vi "DAC trigger.vi"() -> ()   [LabVIEW 2020]
uses:
  <vilib>/DAQmx/configure/timing.llb/DAQmx Timing (Implicit).vi
  <resource>/objmgr/daqmx.rc
  <vilib>/DAQmx/create/channels.llb/DAQmx Create Channel (AO-Voltage-Basic).vi
  <vilib>/Utility/file.llb/Read Delimited Spreadsheet (DBL).vi
  <vilib>/DAQmx/write.llb/DAQmx Write (Analog 1D DBL 1Chan NSamp).vi
  <vilib>/DAQmx/configure/timing.llb/DAQmx Timing (Sample Clock).vi
  <vilib>/DAQmx/create/channels.llb/DAQmx Create Channel (CO-Pulse Generation-Frequency).vi
panel:
  out "Numeric":i32
  in  "Add flyback to polynomial":dbl[](graph)=array[10000 elements]
  in  "File to read":path=path "C:/Users/Hannah/Downloads/newcalibration_voice coil input_25msflyback.txt"
  out "# Samples written per channel":u32=1000
  out "actual frequency":dbl=1000.0
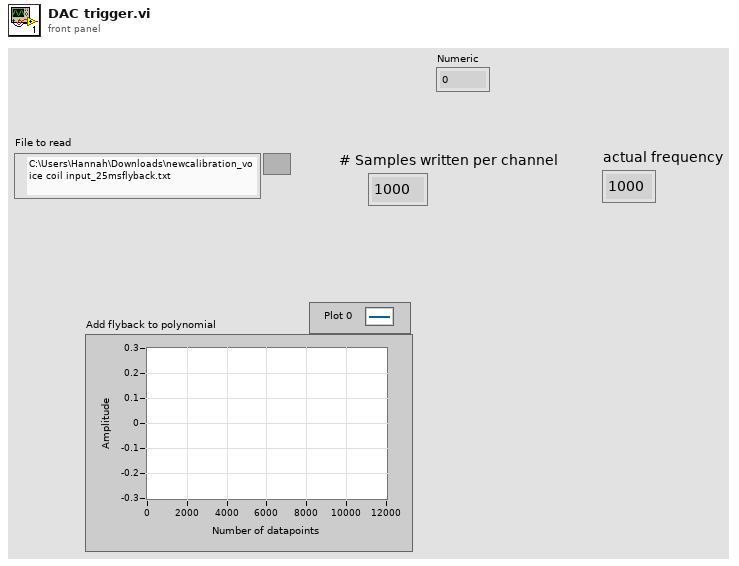
[diagram p1: front panel]
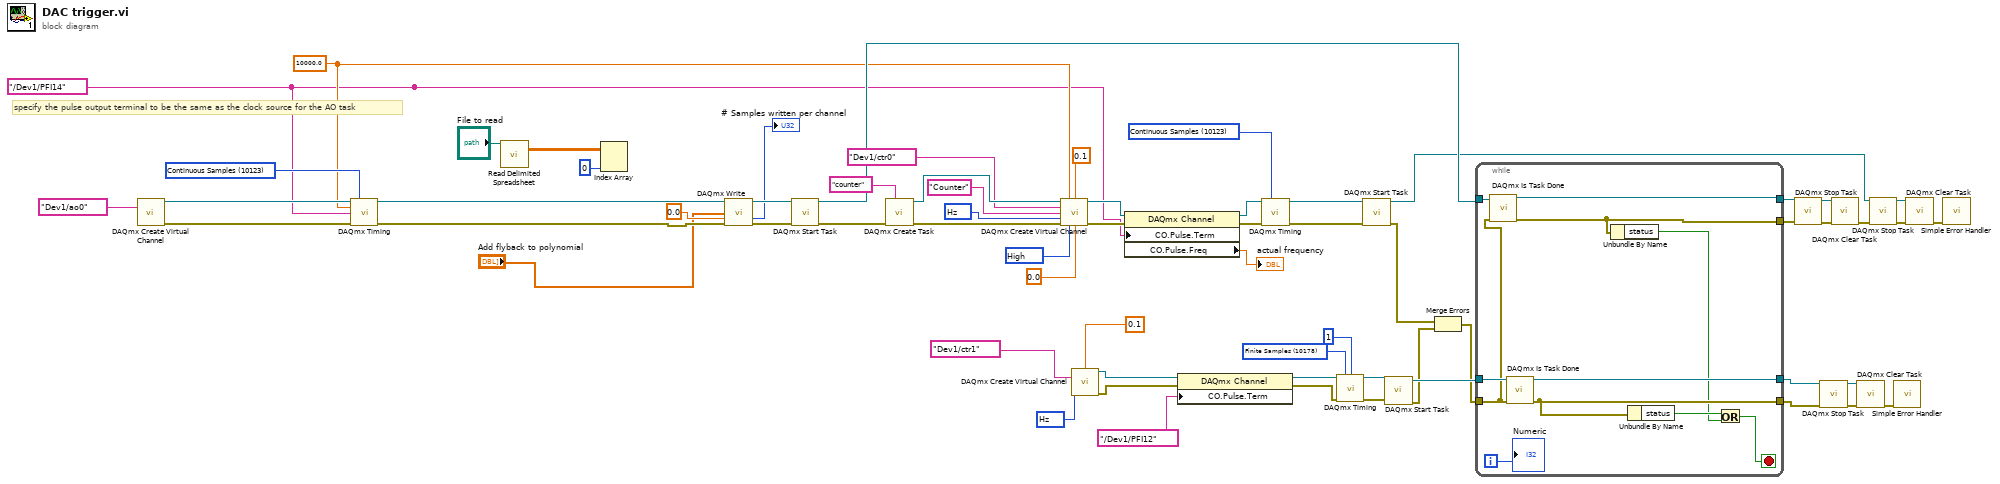
[diagram p0: block diagram]
diagram:
  w2 = 10373 items=["Hz"=10373] ("units")
  w21 = 10178 items=["Finite Samples"=10178, "Continuous Samples"=10123, "Hardware Timed Single Point"=12522] ("sample mode")
  w42 = 10192 items=["High"=10192, "Low"=10214] ("idle state")
  w43 = 10373 items=["Hz"=10373] ("units")
  w18 = tag "/Dev1/PFI14" ("CO.Pulse.Term")
  w31 = 10123 items=["Finite Samples"=10178, "Continuous Samples"=10123, "Hardware Timed Single Point"=12522] ("sample mode")
  w30 = 10000.0 ("rate")
  w63 = 10123 items=["Finite Samples"=10178, "Continuous Samples"=10123, "Hardware Timed Single Point"=12522] ("sample mode")
  # "specify the pulse output terminal to be the same as the clock source for the AO task"
  n1 = call-poly <vilib>:"DAQmx Create Virtual Channel.vi"("physical channels"=tag "Dev1/ao0") -> ("task out"=w65:refnum<k21>, "error out"=w64:errorcluster)  [unwired: 13 in]
  n2 = call-poly <vilib>:"DAQmx Timing.vi"("task/channels in"=w65, "sample mode"=w63, "rate"=w30, "source"=w18, "error in"=w64) -> ("task out"=w34:refnum<k21>, "error out"=w33:errorcluster)  [unwired: 9 in]
  n3 = call-poly <vilib>:"Read Delimited Spreadsheet.vi"("file path (dialog if empty)"="File to read") -> ("all rows"=w37:dbl[][])  [unwired: 9 in, 5 out]
  n4 = Index Array(array=w37, index (col)=0 ("disabled index (col)")) -> ()  [unwired: 1 in, 1 out]
  n5 = call-poly <vilib>:"DAQmx Write.vi"("task/channels in"=w34, "data"="Add flyback to polynomial", "timeout"=0.0, "error in"=w33) -> ("task out"=w48:refnum<k21>, "number of samples written per channel"=→"# Samples written per channel":u32, "error out"=w47:errorcluster)  [unwired: 9 in]
  n6 = call <vilib>:"DAQmx Start Task.vi"("task/channels in"=w48, "error in"=w47) -> ("task out"=w41:refnum<k21>, "error out"=w40:errorcluster)  [unwired: 12 in]
  n7 = call <vilib>:"DAQmx Create Task.vi"("new task name"="counter", "error in"=w40) -> ("task out"=w58:refnum<k21>, "error out"=w56:errorcluster)  [unwired: 12 in]
  n8 = call-poly <vilib>:"DAQmx Create Virtual Channel.vi"("task in"=w58, "frequency"=w30, "duty cycle"=0.1, "counter"=tag "Dev1/ctr0", "name to assign"="Counter", "units"=w43, "error in"=w56, "idle state"=w42, "initial delay"=0.0) -> ("task out"=w55:refnum<k21>, "error out"=w54:errorcluster)  [unwired: 5 in]
  n9 = call-poly <vilib>:"DAQmx Create Virtual Channel.vi"("duty cycle"=0.1, "counter"=tag "Dev1/ctr1", "units"=w2) -> ("task out"=w29:refnum<k21>, "error out"=w28:errorcluster)  [unwired: 11 in]
  n10 = property class="DAQmx Channel"(reference=w55, error in=w54, "CO.Pulse.Term"=w18) -> (reference out=w51:refnum<k21>, error out=w52:errorcluster, "CO.Pulse.Freq"=→"actual frequency":dbl)
  n11 = property class="DAQmx Channel"(reference=w29, error in=w28, "CO.Pulse.Term"=tag "/Dev1/PFI12") -> (reference out=w23:refnum<k21>, error out=w22:errorcluster)
  n12 = call-poly <vilib>:"DAQmx Timing.vi"("task/channels in"=w51, "sample mode"=w31, "error in"=w52) -> ("task out"=w61:refnum<k21>, "error out"=w60:errorcluster)  [unwired: 11 in]
  n13 = call-poly <vilib>:"DAQmx Timing.vi"("task/channels in"=w23, "sample mode"=w21, "samples per channel"=1, "error in"=w22) -> ("task out"=w20:refnum<k21>, "error out"=w19:errorcluster)  [unwired: 10 in]
  n14 = call <vilib>:"DAQmx Start Task.vi"("task/channels in"=w61, "error in"=w60) -> ("task out"=w35:refnum<k21>, "error out"=w5:errorcluster)  [unwired: 12 in]
  n15 = call <vilib>:"DAQmx Start Task.vi"("task/channels in"=w20, "error in"=w19) -> ("task out"=w26:refnum<k21>, "error out"=w4:errorcluster)  [unwired: 12 in]
  n16 = Merge Errors(w5, w4) -> (w3:errorcluster)
  n17 = while {
    tunnel: [w76] -> w50
    tunnel: w41 -> [w74]
    tunnel: [w75] -> w49
    tunnel: w26 -> [w73]
    tunnel: [w72] -> w25
    tunnel: w3 -> [w69]
    tunnel: [w71] -> w24
    i -> [w66]
    stop <- w68 stop-if-true
    n18 = call <vilib>:"DAQmx Is Task Done.vi"("task/channels in"=w74, "error in"=w69) -> ("task out"=w75:refnum<k21>, "error out"=w76:errorcluster)  [unwired: 11 in, 1 out]
    n19 = call <vilib>:"DAQmx Is Task Done.vi"("task/channels in"=w73, "error in"=w69) -> ("task out"=w72:refnum<k21>, "error out"=w71:errorcluster)  [unwired: 11 in, 1 out]
    n20 = Unbundle By Name(w76) -> ("status"=w67:bool)
    n21 = Unbundle By Name(w71) -> ("status"=w70:bool)
    n22 = Or(x=w70, y=w67) -> (x .or. y?=w68:bool)
    "Numeric" <- w66
  }
  n23 = call <vilib>:"DAQmx Stop Task.vi"("task/channels in"=w49, "error in"=w50) -> ("task out"=w12:refnum<k21>, "error out"=w11:errorcluster)  [unwired: 12 in]
  n24 = call <vilib>:"DAQmx Stop Task.vi"("task/channels in"=w25, "error in"=w24) -> ("task out"=w7:refnum<k21>, "error out"=w8:errorcluster)  [unwired: 12 in]
  n25 = call <vilib>:"DAQmx Clear Task.vi"("task in"=w12, "error in"=w11) -> ("error out"=w9:errorcluster)  [unwired: 13 in]
  n26 = call <vilib>:"DAQmx Clear Task.vi"("task in"=w7, "error in"=w8) -> ("error out"=w6:errorcluster)  [unwired: 13 in]
  n27 = call <vilib>:"DAQmx Stop Task.vi"("task/channels in"=w35, "error in"=w9) -> ("task out"=w13:refnum<k21>, "error out"=w14:errorcluster)  [unwired: 12 in]
  n28 = call <vilib>:"Simple Error Handler.vi"("error in (no error)"=w6) -> ()  [unwired: 4 in, 5 out]
  n29 = call <vilib>:"DAQmx Clear Task.vi"("task in"=w13, "error in"=w14) -> ("error out"=w10:errorcluster)  [unwired: 13 in]
  n30 = call <vilib>:"Simple Error Handler.vi"("error in (no error)"=w10) -> ()  [unwired: 4 in, 5 out]
